vi "ReadControlSettings.vi"(8 "error in (no error)":errorcluster, 11 "VI Refnum":refnum<vi>) -> (0 "error out":errorcluster)   [LabVIEW 2013, in "main.lvlib"]
uses:
  main.lvlib
  <vilib>/Utility/config.llb/NI_LVConfig.lvlib
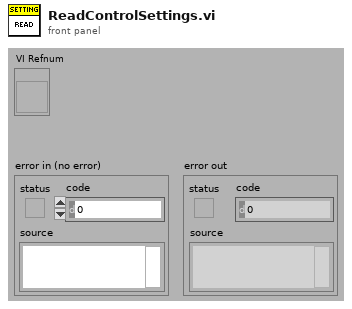
[diagram p1: front panel]
types:
  T1 = typedef "NI_LVConfig.lvlib/Config Data RefNum.ctl" = refnum<k1>
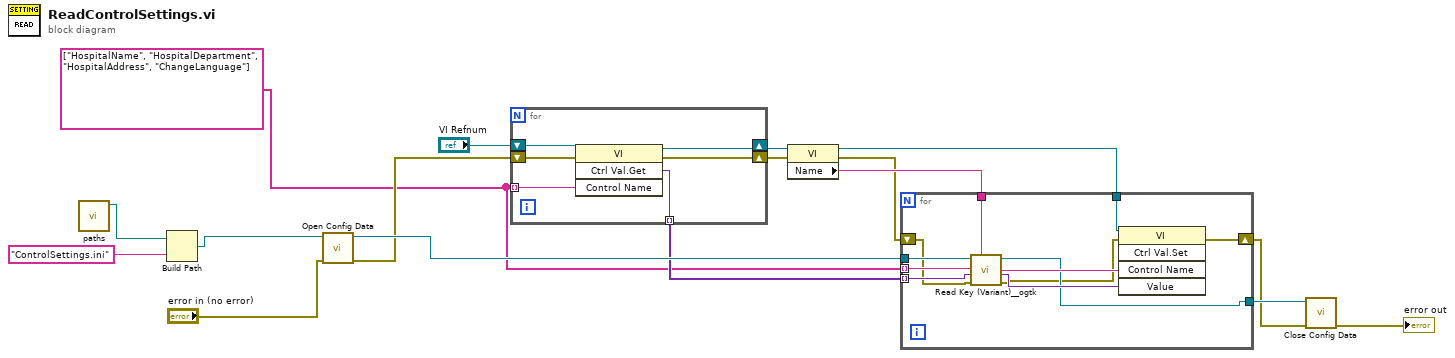
[diagram p0: block diagram]
diagram:
  w2 = string[] ["HospitalName", "HospitalDepartment", "HospitalAddress", "ChangeLanguage"]
  n1 = call "paths.vi"() -> ("PubAppData"=w1:path)  [unwired: 8 in, 3 out]
  n2 = Build Path(base path=w1, name or relative path="ControlSettings.ini") -> (appended path=w11:path)
  n3 = call <vilib>:"Open Config Data.vi"("error in (no error)"="error in (no error)", "configuration file path"=w11) -> ("error out"=w6:errorcluster, "refnum"=w10:T1)  [unwired: 7 in, 1 out]
  n4 = for {
    shift-right: [w23] -> w16
    shift-left: "VI Refnum" -> [w21]
    shift-right: [w22] -> w15
    shift-left: w6 -> [w20]
    tunnel: w2 -> [w19] mode=indexing
    tunnel: [w18] -> w9 mode=indexing
    n5 = invoke class="VI" method="Ctrl Val.Get"(reference=w21, error in=w20, "Control Name"=w19) -> (reference out=w23:refnum<vi>, error out=w22:errorcluster, "Get Control Value Variant"=w18:variant)  [unwired: 1 in, 1 out]
  }
  n6 = property class="VI"(reference=w16, error in=w15) -> (reference out=w13:refnum<vi>, error out=w5:errorcluster, "Name"=w12:string)
  n7 = for {
    tunnel: w13 -> [w33]
    shift-right: [w32] -> w4
    shift-left: w5 -> [w25]
    tunnel: w12 -> [w31]
    tunnel: w10 -> [w30]
    tunnel: w2 -> [w27] mode=indexing
    tunnel: w9 -> [w29] mode=indexing
    tunnel: [w26] -> w8
    n8 = call <userlib>:"Read Key (Variant)__ogtk.vi"("section"=w31, "error in (no error)"=w25, "type"=w29, "key (optional)"=w27, "refnum"=w30) -> ("error out"=w24:errorcluster, "key-value"=w28:variant, "refnum out"=w26:T1)  [unwired: 3 in, 1 out]
    n9 = invoke class="VI" method="Ctrl Val.Set"(reference=w33, error in=w24, "Control Name"=w27, "Value"=w28) -> (error out=w32:errorcluster)  [unwired: 1 in, 4 out]
  }
  n10 = call <vilib>:"Close Config Data.vi"("error in (no error)"=w4, "refnum"=w8) -> ("error out"=→"error out":errorcluster)  [unwired: 8 in, 1 out]
